vi "datatable.vi"(11 "Data Interface in":T1) -> (2 "Value String":string, 3 "Boolean":bool)   [LabVIEW 2013, in "tag bus.lvlib" / "data table.lvlib"]
uses:
  table/data table.lvlib
  table/data table.ctl
  tag/tag descriptor.lvclass
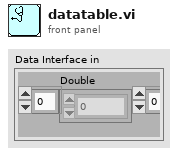
[diagram p1: front panel]
types:
  T1 = typedef "tag bus.lvlib/data table.lvlib/data table.ctl" = cluster{"Double":dbl[], "Single":sgl[], "I64":i64[], "I32":i32[], "I16":i16[], "I8":i8[], "U64":u64[], "U32":u32[], "U16":u16[], "U8":u8[], "Boolean":bool[], "String":string[], "Array of Double":cluster{"DBL Array":dbl[]}[], "Array of Single":cluster{"SGL Array":sgl[]}[], "Array of I64":cluster{"I64 Array":i64[]}[], "Array of I32":cluster{"I32 Array":i32[]}[], "Array of I16":cluster{"I16 Array":i16[]}[], "Array of I8":cluster{"I8 Array":i8[]}[], "Array of U64":cluster{"U64 Array":u64[]}[], "Array of U32":cluster{"U32 Array":u32[]}[], "Array of U16":cluster{"U16 Array":u16[]}[], "Array of U8":cluster{"U8 Array":u8[]}[], "Array of Boolean":cluster{"Boolean Array":bool[]}[], "Array of String":cluster{"String Array":string[]}[]}
  T2 = typedef "tag bus.lvlib/tag descriptor.lvclass/Data Type.ctl" = enum16{"Double", "Single", "I64", "I32", "I16", "I8", "U64", "U32", "U16", "U8", "Boolean", "String", "Array of Double", "Array of Single", "Array of I64", "Array of I32", "Array of I16", "Array of I8", "Array of U64", "Array of U32", "Array of U16", "Array of U8", "Array of Boolean", "Array of String"}
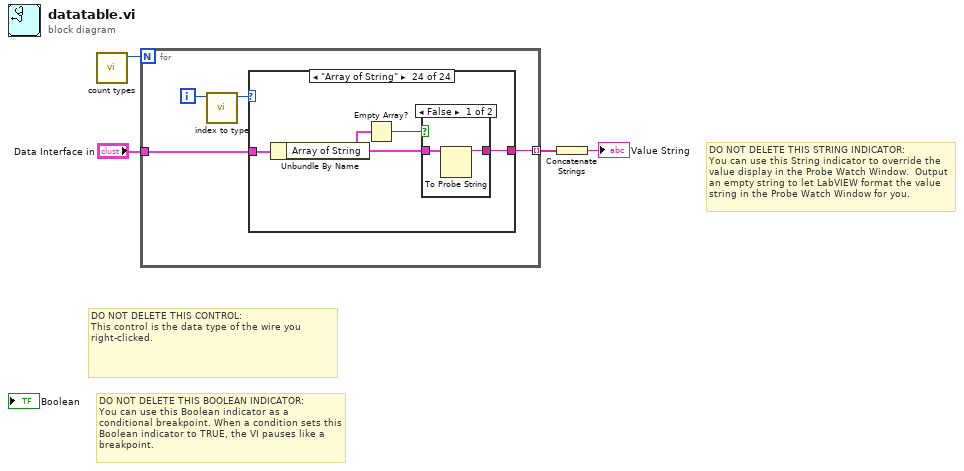
[diagram p0: block diagram]
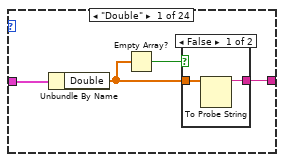
[diagram p2: hidden frame]
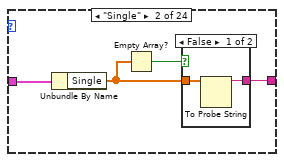
[diagram p4: hidden frame]
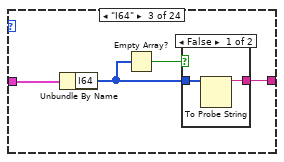
[diagram p6: hidden frame]
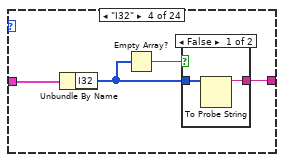
[diagram p8: hidden frame]
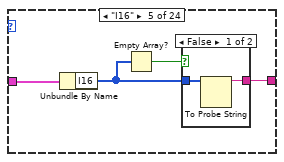
[diagram p10: hidden frame]
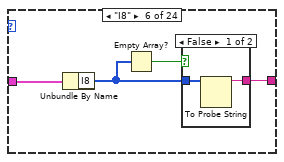
[diagram p12: hidden frame]
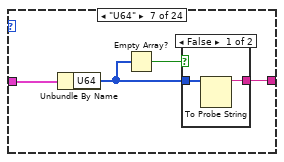
[diagram p14: hidden frame]
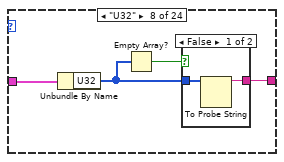
[diagram p16: hidden frame]
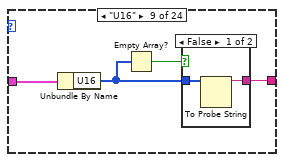
[diagram p18: hidden frame]
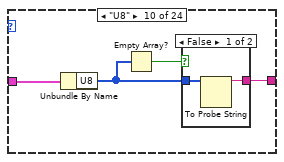
[diagram p20: hidden frame]
diagram:
  # "DO NOT DELETE THIS STRING INDICATOR: \nYou can use this String indicator to override the value display in the Probe Watch Window.  Output an empty string to let LabVIEW format the value string in the Probe Watch Window for you."
  # "DO NOT DELETE THIS BOOLEAN INDICATOR: \nYou can use this Boolean indicator as a conditional breakpoint. When a condition sets this Boolean indicator to TRUE, the VI pauses like a breakpoint."
  # "DO NOT DELETE THIS CONTROL: \nThis control is the data type of the wire you right-clicked."
  n1 = call "count types.vi"() -> ("type count"=w4:i32)  [unwired: 11 in]
  n2 = for {
    N: w4 -> [_]
    tunnel: "Data Interface in" -> [w7]
    tunnel: [w5] -> w2 mode=indexing
    i -> [w8]
    n3 = call "index to type.vi"("I32"=w8) -> ("type"=w6:T2)  [unwired: 10 in]
    n4 = case shown="\"Array of String\"" w6 {
      tunnel: w7 -> [w12 w18 w24 w30 w36 w42 w48 w54 w60 w66 w72 w78 w84 w90 w96 w102 w108 w114 w120 w126 w132 w138 w144 w150]
      tunnel: [w9 w15 w21 w27 w33 w39 w45 w51 w57 w63 w69 w75 w81 w87 w93 w99 w105 w111 w117 w123 w129 w135 w141 w147] -> w5
      frame "Double" {
        n5 = Unbundle By Name(w12) -> ("Double"=w10:dbl[])
        n6 = Empty Array?(array=w10) -> (empty?=w11:bool)
        n7 = case shown="False" w11 {
          tunnel: w10 -> [w14 _]
          tunnel: [w13 _] -> w9
          frame False {
            n8 = To Probe String(7:w14) -> (3:w13:string)  [unwired: 2 in, 1 out]
          }
          frame True {
          }
        }
      }
      frame "Single" {
        n9 = Unbundle By Name(w18) -> ("Single"=w16:sgl[])
        n10 = Empty Array?(array=w16) -> (empty?=w17:bool)
        n11 = case shown="False" w17 {
          tunnel: w16 -> [w20 _]
          tunnel: [w19 _] -> w15
          frame False {
            n12 = To Probe String(7:w20) -> (3:w19:string)  [unwired: 2 in, 1 out]
          }
          frame True {
          }
        }
      }
      frame "I64" {
        n13 = Unbundle By Name(w24) -> ("I64"=w22:i64[])
        n14 = Empty Array?(array=w22) -> (empty?=w23:bool)
        n15 = case shown="False" w23 {
          tunnel: w22 -> [w26 _]
          tunnel: [w25 _] -> w21
          frame False {
            n16 = To Probe String(7:w26) -> (3:w25:string)  [unwired: 2 in, 1 out]
          }
          frame True {
          }
        }
      }
      frame "I32" {
        n17 = Unbundle By Name(w30) -> ("I32"=w28:i32[])
        n18 = Empty Array?(array=w28) -> (empty?=w29:bool)
        n19 = case shown="False" w29 {
          tunnel: w28 -> [w32 _]
          tunnel: [w31 _] -> w27
          frame False {
            n20 = To Probe String(7:w32) -> (3:w31:string)  [unwired: 2 in, 1 out]
          }
          frame True {
          }
        }
      }
      frame "I16" {
        n21 = Unbundle By Name(w36) -> ("I16"=w34:i16[])
        n22 = Empty Array?(array=w34) -> (empty?=w35:bool)
        n23 = case shown="False" w35 {
          tunnel: w34 -> [w38 _]
          tunnel: [w37 _] -> w33
          frame False {
            n24 = To Probe String(7:w38) -> (3:w37:string)  [unwired: 2 in, 1 out]
          }
          frame True {
          }
        }
      }
      frame "I8" {
        n25 = Unbundle By Name(w42) -> ("I8"=w40:i8[])
        n26 = Empty Array?(array=w40) -> (empty?=w41:bool)
        n27 = case shown="False" w41 {
          tunnel: w40 -> [w44 _]
          tunnel: [w43 _] -> w39
          frame False {
            n28 = To Probe String(7:w44) -> (3:w43:string)  [unwired: 2 in, 1 out]
          }
          frame True {
          }
        }
      }
      frame "U64" {
        n29 = Unbundle By Name(w48) -> ("U64"=w46:u64[])
        n30 = Empty Array?(array=w46) -> (empty?=w47:bool)
        n31 = case shown="False" w47 {
          tunnel: w46 -> [w50 _]
          tunnel: [w49 _] -> w45
          frame False {
            n32 = To Probe String(7:w50) -> (3:w49:string)  [unwired: 2 in, 1 out]
          }
          frame True {
          }
        }
      }
      frame "U32" {
        n33 = Unbundle By Name(w54) -> ("U32"=w52:u32[])
        n34 = Empty Array?(array=w52) -> (empty?=w53:bool)
        n35 = case shown="False" w53 {
          tunnel: w52 -> [w56 _]
          tunnel: [w55 _] -> w51
          frame False {
            n36 = To Probe String(7:w56) -> (3:w55:string)  [unwired: 2 in, 1 out]
          }
          frame True {
          }
        }
      }
      frame "U16" {
        n37 = Unbundle By Name(w60) -> ("U16"=w58:u16[])
        n38 = Empty Array?(array=w58) -> (empty?=w59:bool)
        n39 = case shown="False" w59 {
          tunnel: w58 -> [w62 _]
          tunnel: [w61 _] -> w57
          frame False {
            n40 = To Probe String(7:w62) -> (3:w61:string)  [unwired: 2 in, 1 out]
          }
          frame True {
          }
        }
      }
      frame "U8" {
        n41 = Unbundle By Name(w66) -> ("U8"=w64:u8[])
        n42 = Empty Array?(array=w64) -> (empty?=w65:bool)
        n43 = case shown="False" w65 {
          tunnel: w64 -> [w68 _]
          tunnel: [w67 _] -> w63
          frame False {
            n44 = To Probe String(7:w68) -> (3:w67:string)  [unwired: 2 in, 1 out]
          }
          frame True {
          }
        }
      }
      frame "Boolean" {
        n45 = Unbundle By Name(w72) -> ("Boolean"=w70:bool[])
        n46 = Empty Array?(array=w70) -> (empty?=w71:bool)
        n47 = case shown="False" w71 {
          tunnel: w70 -> [w74 _]
          tunnel: [w73 _] -> w69
          frame False {
            n48 = To Probe String(7:w74) -> (3:w73:string)  [unwired: 2 in, 1 out]
          }
          frame True {
          }
        }
      }
      frame "String" {
        n49 = Unbundle By Name(w78) -> ("String"=w76:string[])
        n50 = Empty Array?(array=w76) -> (empty?=w77:bool)
        n51 = case shown="False" w77 {
          tunnel: w76 -> [w80 _]
          tunnel: [w79 _] -> w75
          frame False {
            n52 = To Probe String(7:w80) -> (3:w79:string)  [unwired: 2 in, 1 out]
          }
          frame True {
          }
        }
      }
      frame "Array of Double" {
        n53 = Unbundle By Name(w84) -> ("Array of Double"=w82:cluster{"DBL Array":dbl[]}[])
        n54 = Empty Array?(array=w82) -> (empty?=w83:bool)
        n55 = case shown="False" w83 {
          tunnel: w82 -> [w86 _]
          tunnel: [w85 _] -> w81
          frame False {
            n56 = To Probe String(7:w86) -> (3:w85:string)  [unwired: 2 in, 1 out]
          }
          frame True {
          }
        }
      }
      frame "Array of Single" {
        n57 = Unbundle By Name(w90) -> ("Array of Single"=w88:cluster{"SGL Array":sgl[]}[])
        n58 = Empty Array?(array=w88) -> (empty?=w89:bool)
        n59 = case shown="False" w89 {
          tunnel: w88 -> [w92 _]
          tunnel: [w91 _] -> w87
          frame False {
            n60 = To Probe String(7:w92) -> (3:w91:string)  [unwired: 2 in, 1 out]
          }
          frame True {
          }
        }
      }
      frame "Array of I64" {
        n61 = Unbundle By Name(w96) -> ("Array of I64"=w94:cluster{"I64 Array":i64[]}[])
        n62 = Empty Array?(array=w94) -> (empty?=w95:bool)
        n63 = case shown="False" w95 {
          tunnel: w94 -> [w98 _]
          tunnel: [w97 _] -> w93
          frame False {
            n64 = To Probe String(7:w98) -> (3:w97:string)  [unwired: 2 in, 1 out]
          }
          frame True {
          }
        }
      }
      frame "Array of I32" {
        n65 = Unbundle By Name(w102) -> ("Array of I32"=w100:cluster{"I32 Array":i32[]}[])
        n66 = Empty Array?(array=w100) -> (empty?=w101:bool)
        n67 = case shown="False" w101 {
          tunnel: w100 -> [w104 _]
          tunnel: [w103 _] -> w99
          frame False {
            n68 = To Probe String(7:w104) -> (3:w103:string)  [unwired: 2 in, 1 out]
          }
          frame True {
          }
        }
      }
      frame "Array of I16" {
        n69 = Unbundle By Name(w108) -> ("Array of I16"=w106:cluster{"I16 Array":i16[]}[])
        n70 = Empty Array?(array=w106) -> (empty?=w107:bool)
        n71 = case shown="False" w107 {
          tunnel: w106 -> [w110 _]
          tunnel: [w109 _] -> w105
          frame False {
            n72 = To Probe String(7:w110) -> (3:w109:string)  [unwired: 2 in, 1 out]
          }
          frame True {
          }
        }
      }
      frame "Array of I8" {
        n73 = Unbundle By Name(w114) -> ("Array of I8"=w112:cluster{"I8 Array":i8[]}[])
        n74 = Empty Array?(array=w112) -> (empty?=w113:bool)
        n75 = case shown="False" w113 {
          tunnel: w112 -> [w116 _]
          tunnel: [w115 _] -> w111
          frame False {
            n76 = To Probe String(7:w116) -> (3:w115:string)  [unwired: 2 in, 1 out]
          }
          frame True {
          }
        }
      }
      frame "Array of U64" {
        n77 = Unbundle By Name(w120) -> ("Array of U64"=w118:cluster{"U64 Array":u64[]}[])
        n78 = Empty Array?(array=w118) -> (empty?=w119:bool)
        n79 = case shown="False" w119 {
          tunnel: w118 -> [w122 _]
          tunnel: [w121 _] -> w117
          frame False {
            n80 = To Probe String(7:w122) -> (3:w121:string)  [unwired: 2 in, 1 out]
          }
          frame True {
          }
        }
      }
      frame "Array of U32" {
        n81 = Unbundle By Name(w126) -> ("Array of U32"=w124:cluster{"U32 Array":u32[]}[])
        n82 = Empty Array?(array=w124) -> (empty?=w125:bool)
        n83 = case shown="False" w125 {
          tunnel: w124 -> [w128 _]
          tunnel: [w127 _] -> w123
          frame False {
            n84 = To Probe String(7:w128) -> (3:w127:string)  [unwired: 2 in, 1 out]
          }
          frame True {
          }
        }
      }
      frame "Array of U16" {
        n85 = Unbundle By Name(w132) -> ("Array of U16"=w130:cluster{"U16 Array":u16[]}[])
        n86 = Empty Array?(array=w130) -> (empty?=w131:bool)
        n87 = case shown="False" w131 {
          tunnel: w130 -> [w134 _]
          tunnel: [w133 _] -> w129
          frame False {
            n88 = To Probe String(7:w134) -> (3:w133:string)  [unwired: 2 in, 1 out]
          }
          frame True {
          }
        }
      }
      frame "Array of U8" {
        n89 = Unbundle By Name(w138) -> ("Array of U8"=w136:cluster{"U8 Array":u8[]}[])
        n90 = Empty Array?(array=w136) -> (empty?=w137:bool)
        n91 = case shown="False" w137 {
          tunnel: w136 -> [w140 _]
          tunnel: [w139 _] -> w135
          frame False {
            n92 = To Probe String(7:w140) -> (3:w139:string)  [unwired: 2 in, 1 out]
          }
          frame True {
          }
        }
      }
      frame "Array of Boolean" {
        n93 = Unbundle By Name(w144) -> ("Array of Boolean"=w142:cluster{"Boolean Array":bool[]}[])
        n94 = Empty Array?(array=w142) -> (empty?=w143:bool)
        n95 = case shown="False" w143 {
          tunnel: w142 -> [w146 _]
          tunnel: [w145 _] -> w141
          frame False {
            n96 = To Probe String(7:w146) -> (3:w145:string)  [unwired: 2 in, 1 out]
          }
          frame True {
          }
        }
      }
      frame "Array of String" {
        n97 = Unbundle By Name(w150) -> ("Array of String"=w148:cluster{"String Array":string[]}[])
        n98 = Empty Array?(array=w148) -> (empty?=w149:bool)
        n99 = case shown="False" w149 {
          tunnel: w148 -> [w152 _]
          tunnel: [w151 _] -> w147
          frame False {
            n100 = To Probe String(7:w152) -> (3:w151:string)  [unwired: 2 in, 1 out]
          }
          frame True {
          }
        }
      }
    }
  }
  n101 = Concatenate Strings(w2) -> (→"Value String":string)
